vi "EXA sal Shm Release.vi"(8 "error in (no error)":errorcluster) -> (0 "error out":errorcluster, 3 "function return":i32)   [LabVIEW 2016, in "SALLV_EXA.lvlib"]
doc: "int EXA_salShmRelease();"
uses:
  SALLV_EXA.lvlib
  SALLV_EXA.so
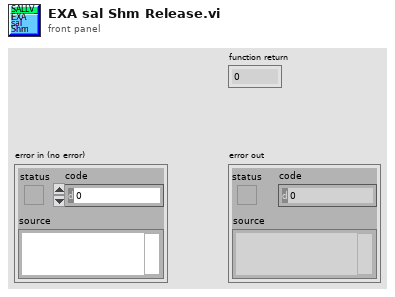
[diagram p1: front panel]
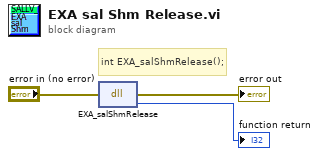
[diagram p0: block diagram]
diagram:
  # "int EXA_salShmRelease();"
  n1 = dll-call lib="home/plotz/SALLV_EXA/SALLV_EXA.*" fn="EXA_salShmRelease"(error in="error in (no error)") -> (error out=→"error out":errorcluster, →"function return":i32)  [unwired: 2 in, 1 out]
